vi "Day 18-Part 2.vi"() -> ()   [LabVIEW 2021]
uses:
  <vilib>/Utility/file.llb/Read Delimited Spreadsheet (string).vi
panel:
  out "Max Magnitude Between any Two Sums":i32
  out "Input":string[](array[string])
  in  "Input File":enum32{"example input", "input"}(radio)
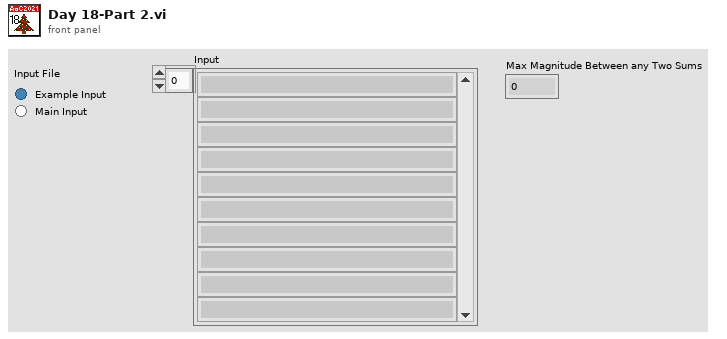
[diagram p1: front panel]
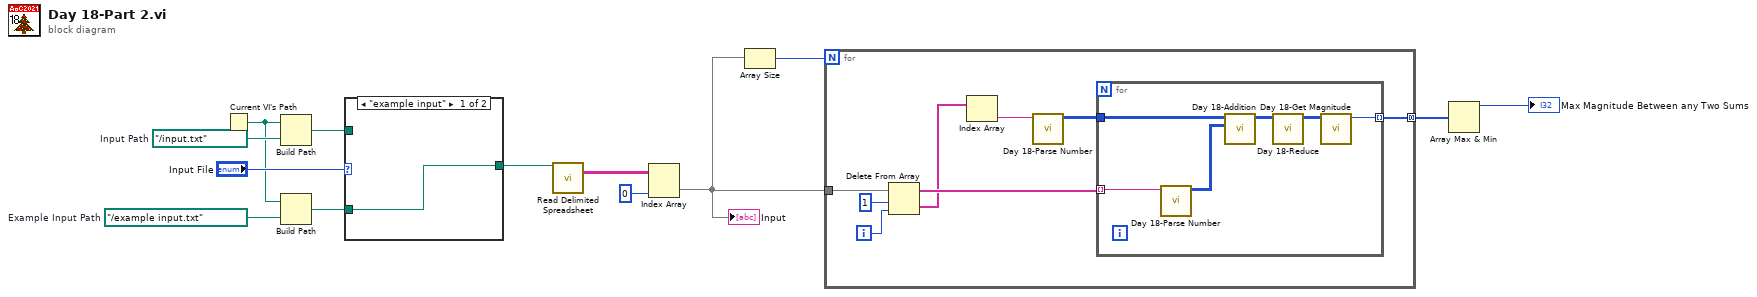
[diagram p0: block diagram]
diagram:
  w12 = path "../example input.txt"  # Example Input Path
  w13 = path "../input.txt"  # Input Path
  n1 = Current VI's Path() -> (path=w7:path)
  n2 = Build Path(base path=w7, name or relative path=w13) -> (appended path=w10:path)
  n3 = Build Path(base path=w7, name or relative path=w12) -> (appended path=w9:path)
  n4 = case shown="\"example input\"" "Input File" {
    tunnel: w10 -> [_ w15]
    tunnel: w9 -> [w14 _]
    tunnel: [w14 w15] -> w8
    frame "example input" {
    }
    frame "input" {
    }
  }
  n5 = call-poly <vilib>:"Read Delimited Spreadsheet.vi"("file path (dialog if empty)"=w8) -> ("all rows"=w6:string[][])  [unwired: 9 in, 5 out]
  n6 = Index Array(array=w6, index (col)=0 ("disabled index (col)")) -> (element=w2:string[])  [unwired: 1 in]
  "Input" <- w2
  n7 = Array Size(array=w2) -> (size(s)=w1:i32)
  n8 = for {
    N: w1 -> [_]
    tunnel: w2 -> [w19]
    tunnel: [w16] -> w4 mode=concatenating
    i -> [w18]
    n9 = Delete From Array(array=w19, length=1, index=w18) -> (deleted portion=w21:string[], array with subset deleted=w22:string[])
    n10 = Index Array(array=w21) -> (element=w20:string)  [unwired: 1 in]
    n11 = call "Day 18-Parse Number.vi"("Data in"=w20) -> ("Data out"=w17:i32[][])  [unwired: 10 in]
    n12 = for {
      tunnel: w22 -> [w29] mode=indexing
      tunnel: w17 -> [w26]
      tunnel: [w25] -> w16 mode=indexing
      n13 = call "Day 18-Parse Number.vi"("Data in"=w29) -> ("Data out"=w28:i32[][])  [unwired: 10 in]
      n14 = call "Day 18-Addition.vi"("Data 2 in"=w28, "Data 1 in"=w26) -> ("Data out"=w27:i32[][])  [unwired: 9 in]
      n15 = call "Day 18-Reduce.vi"("Array in"=w27) -> ("Array out"=w24:i32[][])  [unwired: 10 in]
      n16 = call "Day 18-Get Magnitude.vi"("Array in"=w24) -> ("Magnitude"=w25:i32)  [unwired: 10 in]
    }
  }
  n17 = Array Max & Min(array=w4) -> (max value=→"Max Magnitude Between any Two Sums":i32)  [unwired: 3 out]
